vi "publisher tests Reader 5.vi"() -> ()   [LabVIEW 2018]
uses:
  publisher action.ctl
panel:
  out "Numeric":i32
  in  "read":bool
  out "number":dbl
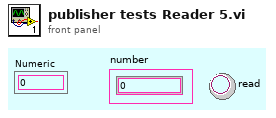
[diagram p1: front panel]
types:
  T1 = typedef "publisher action.ctl" = enum16{"set", "get", "init", "check"}
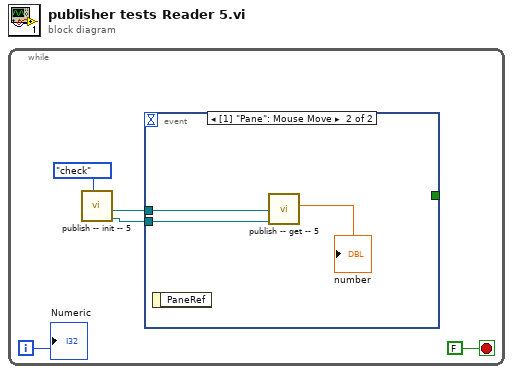
[diagram p0: block diagram]
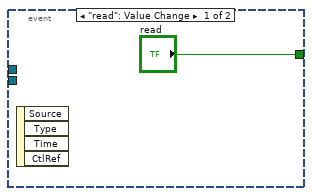
[diagram p2: hidden frame]
diagram:
  n1 = while {
    i -> [w1]
    stop <- FALSE stop-if-true
    n2 = call "publish -- init -- 5.vi"("publisher action"=publisher_action."check") -> ("request event"=w3:refnum<user-event>, "response event"=w2:refnum<user-event>)  [unwired: 9 in]
    n3 = event shown="[1] \"Pane\": Mouse Move" {
      selector: _ -> [_ _]
      dyn-events: _ -> [_ _]
      timeout: _ -> [_ _]
      tunnel: ["read" _] -> _
      tunnel: w2 -> [_ w9]
      tunnel: w3 -> [_ w8]
      event "read": Value Change {
        n4 = event-data() -> ()  [unwired: 1 in, 4 out]
      }
      event Mouse Move {
        n5 = event-data() -> ()  [unwired: 1 in, 1 out]
        n6 = call "publish -- get -- 5.vi"("request event"=w8, "response event"=w9) -> ("nnumber"=→"number":dbl)  [unwired: 9 in]
      }
    }
    "Numeric" <- w1
  }
